vi "M03 Toy factory.vi"(11 "NXT/EV3":T1) -> (1 "Angle out":sgl, 3 "EV3 out":T1)   [LabVIEW 2016]
uses:
  <vilib>/NXT/Subs/LVHSConnector.ctl
  <vilib>/NXT/LegoClasses/BrickReference/BrickReference.lvclass
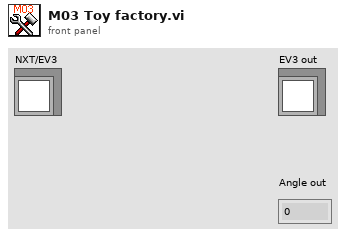
[diagram p1: front panel]
types:
  T1 = typedef "LVHSConnector.ctl" = refnum<class "BrickReference.lvclass">
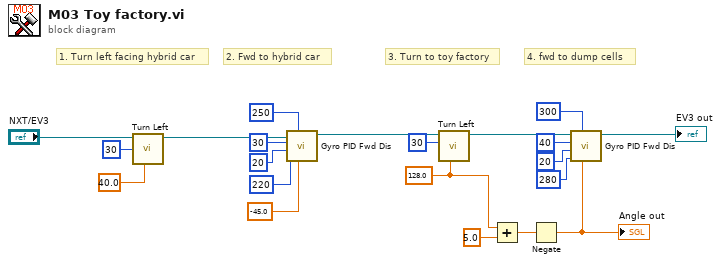
[diagram p0: block diagram]
diagram:
  w4 = sgl 128.0 ("Turning angle")
  # "4. fwd to dump cells"
  # "3. Turn to toy factory"
  # "2. Fwd to hybrid car"
  # "1. Turn left facing hybrid car"
  n1 = call "Turn Left.vi"("Turning angle"=sgl 40.0, "Motor B (right)"=i8 30, "EV3 in"="NXT/EV3") -> ("EV3 out"=w20:T1)  [unwired: 8 in]
  n2 = call "Gyro PID Fwd Dis.vi"("Target angle"=sgl -45.0, "Threshold to stop"=250, "Threshold to slow"=220, "Min. speed"=20, "Max. speed"=30, "EV3 in"=w20) -> ("EV3 out"=w14:T1)  [unwired: 5 in]
  n3 = call "Turn Left.vi"("Turning angle"=w4, "Motor B (right)"=i8 30, "EV3 in"=w14) -> ("EV3 out"=w8:T1)  [unwired: 8 in]
  n4 = Add(x=w4, y=sgl 5.0) -> (x+y=w2:sgl)
  n5 = Negate(x=w2) -> (-x=w1:sgl)
  "Angle out" <- w1
  n6 = call "Gyro PID Fwd Dis.vi"("Target angle"=w1, "Threshold to stop"=300, "Threshold to slow"=280, "Min. speed"=20, "Max. speed"=40, "EV3 in"=w8) -> ("EV3 out"=→"EV3 out":T1)  [unwired: 5 in]
